vi "Destroy.vi"(0 "reference":refnum<class "MultiLineString.lvclass">, 5 "error in (no error)":errorcluster) -> (15 "# of objects":i32, 19 "error out":errorcluster)   [LabVIEW 2014, in "MultiLineString.lvclass"]
doc: "Destroys an object created with a MultiLineString constructor VI or a subclass of the MultiLineString class. This VI must be reentrant.\n\n[GOOP 2.3]"
uses:
  <resource>/Framework/Providers/Open_GDS/UML/MultiLineString_class/MultiLineString.lvclass
panel:
  out "reference out":refnum<class "MultiLineString.lvclass">
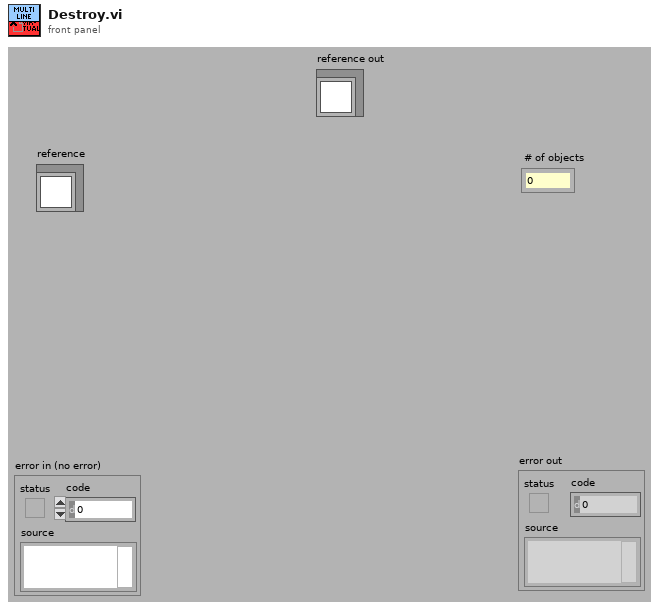
[diagram p1: front panel]
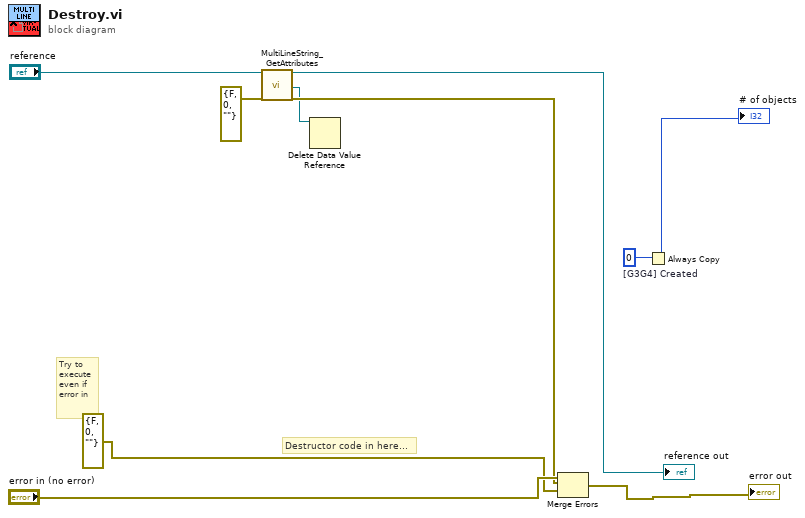
[diagram p0: block diagram]
diagram:
  w1 = 0  # [G3G4] Created
  # "Destructor code in here..."
  # "Try to\nexecute\neven if\nerror in"
  n1 = call <resource>:"MultiLineString_GetAttributes.vi"("reference in"="reference", "error in (no error)"=errorcluster {"status"=FALSE, "code"=0, "source"=""}) -> ("reference out"=→"reference out":refnum<class "MultiLineString.lvclass">, "DataRef"=w3:refnum<data-value>, "error out"=w5:errorcluster)  [unwired: 1 in, 14 out]
  n2 = Delete Data Value Reference(data value reference=w3) -> ()  [unwired: 1 in, 2 out]
  n3 = Merge Errors("error in (no error)", w5, errorcluster {"status"=FALSE, "code"=0, "source"=""} ("error in (no error)")) -> (→"error out":errorcluster)
  n4 = Always Copy(1:w1) -> (0:→"# of objects":i32)
